vi "Overrid Dynamic Dispatch VIs.vi"(8 "error in (no error)":errorcluster, 11 "Mock Class Generator in":refnum<class "Pure Mock Class Generator.lvclass">) -> (0 "error out":errorcluster, 3 "Mock Class Generator out":refnum<class "Pure Mock Class Generator.lvclass">)   [LabVIEW 2020, in "Pure Mock Class Generator.lvclass"]
uses:
  Pure Mock Class Generator.lvclass
  Pure Mock Class Generator.lvclass/Pure Mock Class Generator.ctl
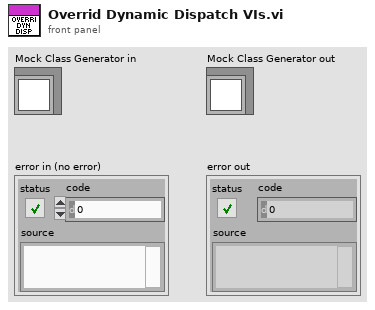
[diagram p1: front panel]
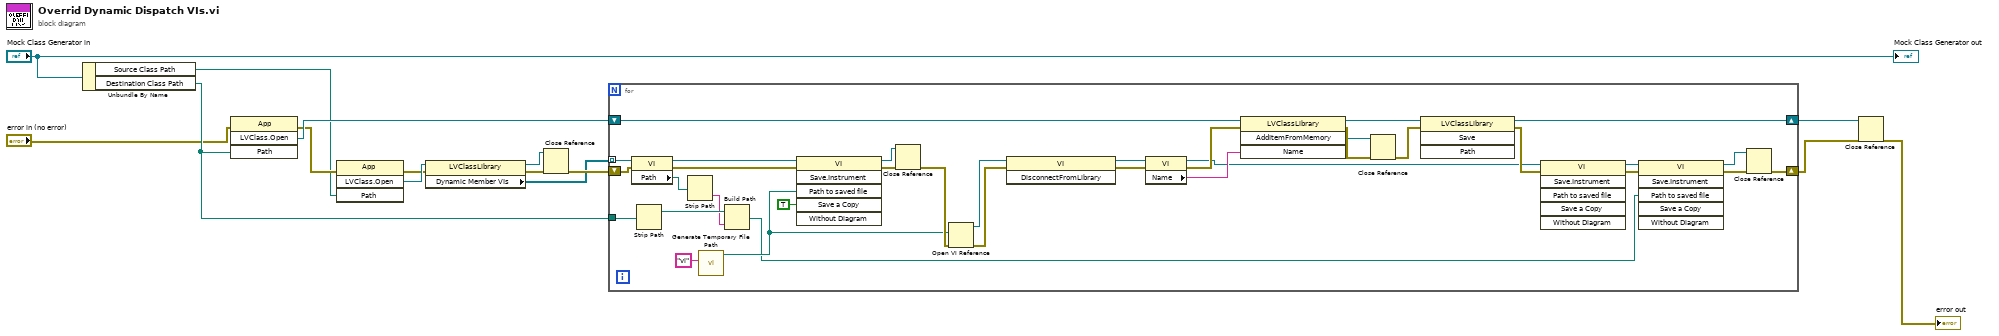
[diagram p0: block diagram]
diagram:
  n1 = Unbundle By Name("Mock Class Generator in") -> ("Source Class Path"=w10:path, "Destination Class Path"=w14:path)
  n2 = invoke class="App" method="LVClass.Open"(error in="error in (no error)", "Path"=w14) -> (error out=w12:errorcluster, "LVClass.Open"=w13:refnum<vi>)  [unwired: 2 in, 2 out]
  n3 = invoke class="App" method="LVClass.Open"(error in=w12, "Path"=w10) -> (error out=w8:errorcluster, "LVClass.Open"=w9:refnum<vi>)  [unwired: 2 in, 2 out]
  n4 = property class="LVClassLibrary"(reference=w9, error in=w8) -> (reference out=w2:refnum<vi>, error out=w3:errorcluster, "Dynamic Member VIs"=w4:refnum<vi>[])
  n5 = Close Reference(reference=w2, error in (no error)=w3) -> (error out=w5:errorcluster)
  n6 = for {
    tunnel: w4 -> [w49] mode=indexing
    shift-right: [w36] -> w6
    shift-left: w5 -> [w43]
    shift-right: [w34] -> w7
    shift-left: w13 -> [w41]
    tunnel: w14 -> [w22]
    n7 = property class="VI"(reference=w49, error in=w43) -> (reference out=w44:refnum<vi>, error out=w42:errorcluster, "Path"=w48:path)
    n8 = Strip Path(path=w22) -> (stripped path=w47:path)  [unwired: 1 out]
    n9 = Strip Path(path=w48) -> (name=w46:string)  [unwired: 1 out]
    n10 = call <vilib>:"Generate Temporary File Path.vi"("Temporary File Extension (tmp)"="vi") -> ("Unique Temporary File Path"=w20:path)  [unwired: 9 in, 1 out]
    n11 = Build Path(base path=w47, name or relative path=w46) -> (appended path=w19:path)
    n12 = invoke class="VI" method="Save.Instrument"(reference=w44, error in=w42, "Path to saved file"=w20, "Save a Copy"=TRUE) -> (reference out=w26:refnum<vi>, error out=w29:errorcluster)  [unwired: 2 in, 4 out]
    n13 = Close Reference(reference=w26, error in (no error)=w29) -> (error out=w25:errorcluster)
    n14 = Open VI Reference(vi path=w20, error in (no error)=w25) -> (vi reference=w24:refnum<vi>, error out=w23:errorcluster)  [unwired: 4 in]
    n15 = invoke class="VI" method="DisconnectFromLibrary"(reference=w24, error in=w23) -> (reference out=w27:refnum<vi>, error out=w28:errorcluster)  [unwired: 1 in, 1 out]
    n16 = property class="VI"(reference=w27, error in=w28) -> (reference out=w17:refnum<vi>, error out=w30:errorcluster, "Name"=w31:string)
    n17 = invoke class="LVClassLibrary" method="AddItemFromMemory"(reference=w41, error in=w30, "Name"=w31) -> (reference out=w35:refnum<vi>, error out=w40:errorcluster, "AddItemFromMemory"=w39:refnum<vi>)  [unwired: 1 in, 1 out]
    n18 = Close Reference(reference=w39, error in (no error)=w40) -> (error out=w33:errorcluster)
    n19 = invoke class="LVClassLibrary" method="Save"(reference=w35, error in=w33) -> (reference out=w34:refnum<vi>, error out=w32:errorcluster)  [unwired: 2 in, 2 out]
    n20 = invoke class="VI" method="Save.Instrument"(reference=w17, error in=w32) -> (reference out=w16:refnum<vi>, error out=w18:errorcluster)  [unwired: 4 in, 4 out]
    n21 = invoke class="VI" method="Save.Instrument"(reference=w16, error in=w18, "Path to saved file"=w19) -> (reference out=w38:refnum<vi>, error out=w37:errorcluster)  [unwired: 3 in, 4 out]
    n22 = Close Reference(reference=w38, error in (no error)=w37) -> (error out=w36:errorcluster)
  }
  n23 = Close Reference(reference=w7, error in (no error)=w6) -> (error out=→"error out":errorcluster)
  "Mock Class Generator out" <- "Mock Class Generator in"
